vi "Autonomous.vi"   [LabVIEW 2015]
doc: "This VI starts when autonomous period begins, and will automatically be terminated when it ends. You can carry out timed or sensor driven operations directly to I/O or to subsystems without needing to return to the caller."
uses:
  <vilib>/Rock Robotics/WPI/Utilities/WPI_GetSetVariantRefNum.vi
types:
  T1 = typedef "WPI_JoystickDevRef.ctl" = cluster{"Device":T2}
  T2 = typedef "WPI_JoystickDeviceEnum.ctl" = enum16{"USB 0", "USB 1", "USB 2", "USB 3", "USB 4", "USB 5"}
  T3 = typedef "Command Status Info.ctl" = cluster{"Name":string, "Status":T4, "notifier out":T5}
  T4 = typedef "Completion Status.ctl" = enum16{"Successful", "Aborted", "Incomplete"}
  T5 = typedef "Completion Notifier.ctl" = refnum<notifier>
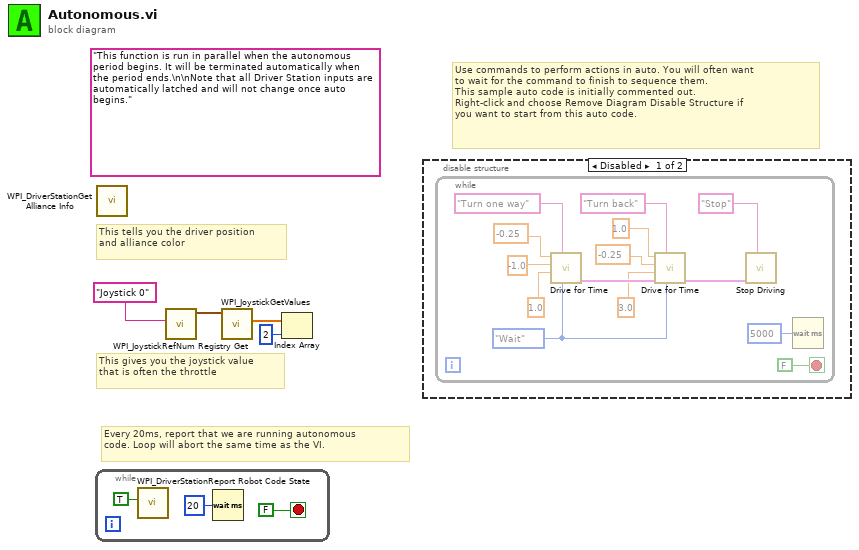
[diagram p0: block diagram]
diagram:
  (unwired) "This function is run in parallel when the autonomous period begins. It will be terminated automatically when the period ends.\n\nNote that all Driver Station inputs are automatically latched and will not change once auto begins."
  # "Every 20ms, report that we are running autonomous\ncode. Loop will abort the same time as the VI."
  # "This gives you the joystick value\nthat is often the throttle"
  # "Use commands to perform actions in auto. You will often want\nto wait for the command to finish to sequence them.\nThis sample auto code is initially commented out. \nRight-click and choose Remove Diagram Disable Structure if\nyou want to start from this auto code."
  # "This tells you the driver position\nand alliance color"
  n1 = while {
    stop <- FALSE stop-if-true
    n2 = call <vilib>:"WPI_DriverStationReport Robot Code State.vi"("Autonomous"=TRUE) -> ()  [unwired: 10 in, 1 out]
    n3 = Wait (ms)(milliseconds to wait=u32 20) -> ()  [unwired: 1 out]
  }
  n4 = call <vilib>:"WPI_DriverStationGet Alliance Info.vi"() -> ()  [unwired: 12 out]
  n5 = call <vilib>:"WPI_JoystickRefNum Registry Get.vi"("refnum name"="Joystick 0") -> ("JoystickDevRef"=w3:T1)  [unwired: 1 in, 9 out]
  n6 = call <vilib>:"WPI_JoystickGetValues.vi"("JoystickDevRef"=w3) -> ("Axes"=w2:dbl[])  [unwired: 6 in, 4 out]
  n7 = Index Array(array=w2, index=2) -> ()  [unwired: 1 out]
  n8 = disable-structure shown="Disabled" {
    frame Disabled {
      n9 = while {
        stop <- FALSE stop-if-true
        w12 = enum16{"Start", "Wait"}."Wait" ("Synchronication")
        n10 = call "Drive for Time.vi"("Synchronization"=w12, "Description"="Turn one way", "Seconds"=1.0 ("Delay (s)"), "Right Speed"=-1.0 ("X axis value"), "Left Speed"=-0.25 ("X axis value")) -> ("Command Info Out"=w21:T3)  [unwired: 5 in, 1 out]
        n11 = call "Drive for Time.vi"("Synchronization"=w12, "Description"="Turn back", "Command Info In"=w21, "Seconds"=3.0 ("Delay (s)"), "Right Speed"=-0.25 ("X axis value"), "Left Speed"=1.0 ("X axis value")) -> ("Command Info Out"=w11:T3)  [unwired: 4 in, 1 out]
        n12 = call "Stop Driving.vi"("Description"="Stop", "Command Info In"=w11) -> ()  [unwired: 9 in, 1 out]
        n13 = Wait (ms)(milliseconds to wait=u32 5000 ("millisecond timer value")) -> ()  [unwired: 1 out]
      }
    }
    frame Enabled {
    }
  }
